vi "subvi_twice_bool_crossing_analyser1.vi"(6 "Action":T1, 11 "Input Bool":bool=TRUE) -> (1 "Last Crossing":bool, 3 "Crossed?":bool=TRUE)   [LabVIEW 2014]
uses:
  typedef_twice_bool_crossing.ctl
  typedef_boolcrossing.ctl
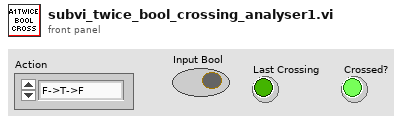
[diagram p1: front panel]
types:
  T1 = typedef "typedef_twice_bool_crossing.ctl" = enum16{"F->T->F", "T->F->T", "Initialise"}
  T2 = typedef "typedef_boolcrossing.ctl" = enum16{"Either", "True-False", "False-True", "Initialise"}
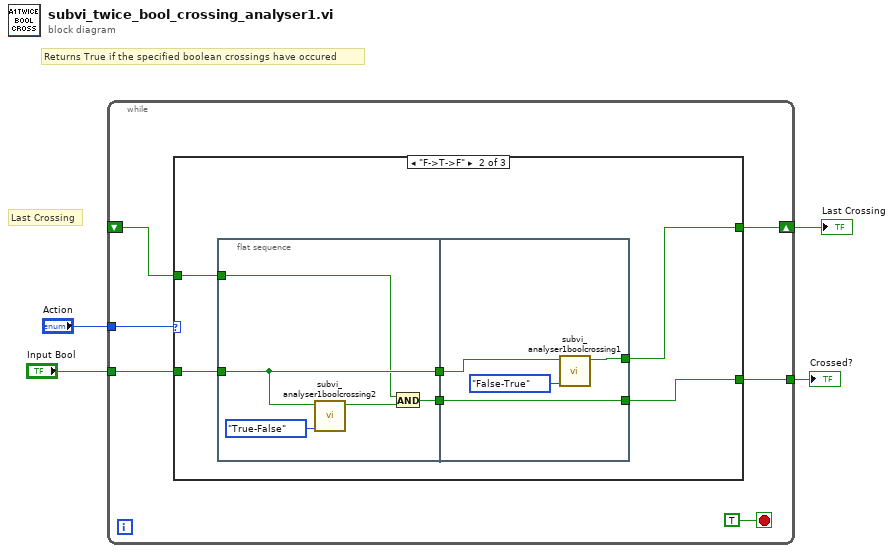
[diagram p0: block diagram]
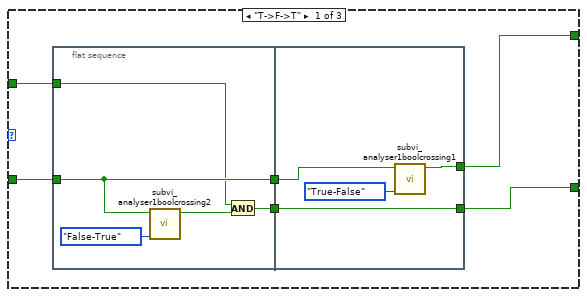
[diagram p2: hidden frame]
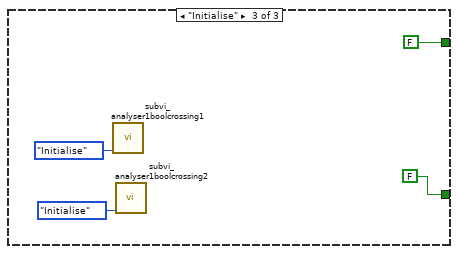
[diagram p3: hidden frame]
diagram:
  # "Last Crossing"
  # "Returns True if the specified boolean crossings have occured"
  n1 = while {
    tunnel: "Action" -> [w10]
    tunnel: "Input Bool" -> [w9]
    shift-right: [w7] -> w1
    shift-left: _ -> [w8]
    tunnel: [w6] -> w2
    stop <- TRUE stop-if-true
    n2 = case shown="\"F->T->F\"" w10 {
      tunnel: w9 -> [w16 w31 _]
      tunnel: w8 -> [w15 w30 _]
      tunnel: [w12 w27 FALSE ("Crossed?")] -> w7
      tunnel: [w11 w26 FALSE ("Crossed?")] -> w6
      frame "T->F->T" {
        n3 = flat-sequence {
          tunnel: w16 -> [w18]
          tunnel: w15 -> [w17]
          tunnel: [w19] -> w14
          tunnel: [w18] -> w13
          tunnel: w14 -> [w22]
          tunnel: w13 -> [w24]
          tunnel: [w23] -> w12
          tunnel: [w22] -> w11
          frame #0 {
            n4 = call "subvi_analyser1boolcrossing2.vi"("Action"=typedef_boolcrossing."False-True", "Input Bool"=w18) -> ("Crossed?"=w20:bool)  [unwired: 9 in]
            n5 = And(x=w17, y=w20) -> (x .and. y?=w19:bool)
          }
          frame #1 {
            n6 = call "subvi_analyser1boolcrossing1.vi"("Action"=typedef_boolcrossing."True-False", "Input Bool"=w24) -> ("Crossed?"=w23:bool)  [unwired: 9 in]
          }
        }
      }
      frame "F->T->F" {
        n7 = flat-sequence {
          tunnel: w31 -> [w33]
          tunnel: w30 -> [w32]
          tunnel: [w34] -> w29
          tunnel: [w33] -> w28
          tunnel: w29 -> [w37]
          tunnel: w28 -> [w39]
          tunnel: [w38] -> w27
          tunnel: [w37] -> w26
          frame #0 {
            n8 = call "subvi_analyser1boolcrossing2.vi"("Action"=typedef_boolcrossing."True-False", "Input Bool"=w33) -> ("Crossed?"=w35:bool)  [unwired: 9 in]
            n9 = And(x=w32, y=w35) -> (x .and. y?=w34:bool)
          }
          frame #1 {
            n10 = call "subvi_analyser1boolcrossing1.vi"("Action"=typedef_boolcrossing."False-True", "Input Bool"=w39) -> ("Crossed?"=w38:bool)  [unwired: 9 in]
          }
        }
      }
      frame "Initialise" {
        n11 = call "subvi_analyser1boolcrossing1.vi"("Action"=typedef_boolcrossing."Initialise") -> ()  [unwired: 10 in, 1 out]
        n12 = call "subvi_analyser1boolcrossing2.vi"("Action"=typedef_boolcrossing."Initialise") -> ()  [unwired: 10 in, 1 out]
      }
    }
  }
  "Crossed?" <- w2
  "Last Crossing" <- w1
